vi "open stop constant.vi"() -> (3 "angle":dbl)   [LabVIEW 2019, in "NeedleValve.lvclass"]
uses:
  NeedleValve.lvclass
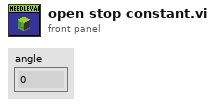
[diagram p1: front panel]
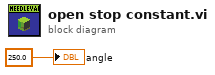
[diagram p0: block diagram]
diagram:
  "angle" <- 250.0 ("y")
